vi "AlliGator Fit Termination Criteria & Quality Metrics Output String.vi"(8 "Error In":errorcluster, 9 "Fit Output":T5={"best nonlinear fit"=[], "best fit parameters"=[], "R^2"=0.0, "RMSE"=0.0, "error out"={"status"=FALSE, "code"=0, "source"=""}, "Fitting Method"=enum."Least Square", "number of function calls"=0, "number of iterations"=0, "covariance"=[], "Chi 2"=0.0, "DOF"=0, "Fit Convergence Criterion"=enum."Continue", "Fitting Algorithm"=enum."Levenberg-Marquardt", "Weighted Fit"=enum."Unweighted", "Gradient"=0.0, "|Delta Chi 2|"=0.0, "|Delta Chi 2|/Chi 2"=0.0, "Max |Delta a| /|a|"=0.0, "Lambda"=0.0, "RSS"=0.0, "AIC"=0.0, "BIC"=0.0, "Max number of function calls"=0, "Max number of iterations"=0, "IRF"={"X Array"=[], "Y Array"=[]}, "IRF Normalization Factor"=0.0, "Decay Normalization Factor"=0.0, "Number of offset fits"=0, "Weighted Chi2"=-1.0, "Unweighted Chi2"=-1.0}, 11 "Termination Criteria":T2) -> (0 "Error Out":errorcluster, 1 "Weighted Fit":T1, 3 "String":string)   [LabVIEW 2021, in "AlliGator Decay Fit.lvlib"]
doc: "Creates a string describing the fit termination criteria and quality metrics."
uses:
  AlliGator Decay Fit.lvlib
  Fits/Nonlinear Fit Method.ctl
  Fits/Fits.lvlib
  <vilib>/Analysis/Matrix/Datatypes/RealMatrix.ctl
  <vilib>/Analysis/Matrix/NI_Matrix.lvlib
  Fits/Convergence Criteria.ctl
  Fits/Non-linear Fitting Algorithm.ctl
  Fits/Non-linear Fit Output v4.ctl
  Graphs/XY Graph/XY Graph Plot Data.ctl
  Graphs/XY Graph/XY Graph Add-Ons.lvlib
  Fits/IRF(X)PSED/Fit Weights Type v2.ctl
panel:
  in  "Fitting Method":T3
  in  "Fitting Algorithm":T4
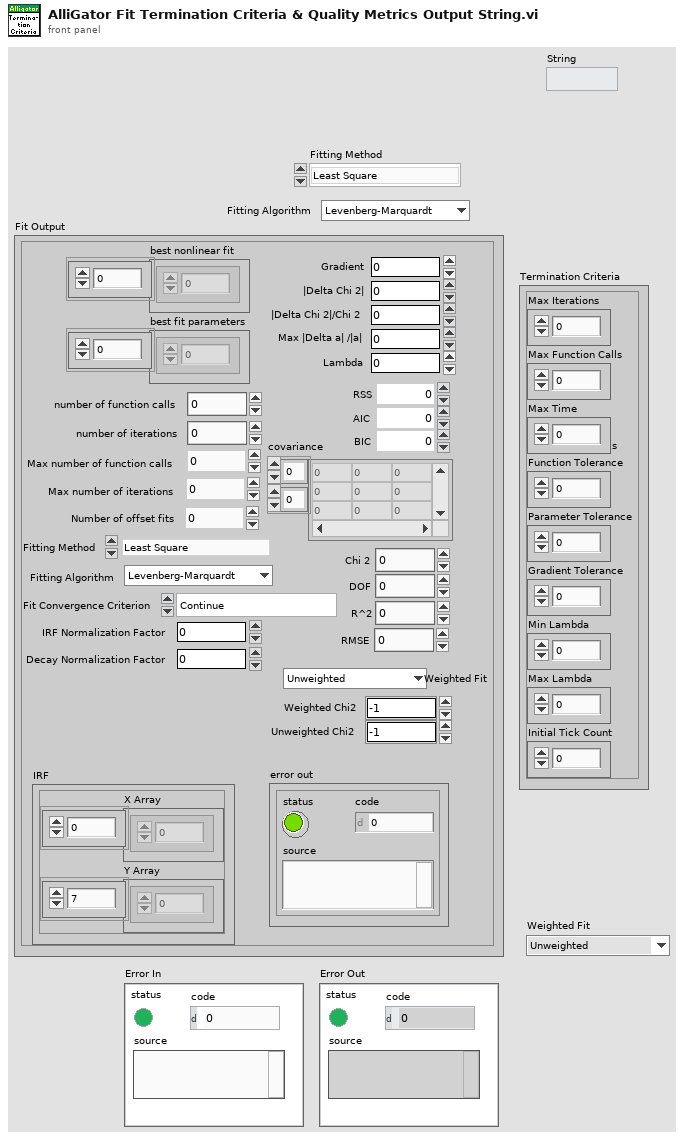
[diagram p1: front panel]
types:
  T1 = typedef "Fits.lvlib/Fit Weights Type v2.ctl" = enum16{"Unweighted", "1/Variance (Neyman)", "1/Variance (Pearson)", "Best of All"}
  T2 = cluster{"Max Iterations":i32, "Max Function Calls":i32, "Max Time":dbl[unit], "Function Tolerance":dbl, "Parameter Tolerance":dbl, "Gradient Tolerance":dbl, "Min Lambda":dbl, "Max Lambda":dbl, "Initial Tick Count":u32}
  T3 = typedef "Fits.lvlib/Nonlinear Fit Method.ctl" = enum16{"Least Square", "Least Absolute Residual", "Bisquare", "MLE"}
  T4 = typedef "Fits.lvlib/Non-linear Fitting Algorithm.ctl" = enum16{"Levenberg-Marquardt", "Trust-Region Dogleg"}
  T5 = typedef "Fits.lvlib/Non-linear Fit Output v4.ctl" = cluster{"best nonlinear fit":dbl[], "best fit parameters":dbl[], "R^2":dbl, "RMSE":dbl, "error out":errorcluster, "Fitting Method":T3, "number of function calls":i32, "number of iterations":i32, "covariance":T6, "Chi 2":dbl, "DOF":i32, "Fit Convergence Criterion":T7, "Fitting Algorithm":T4, "Weighted Fit":T1, "Gradient":dbl, "|Delta Chi 2|":dbl, "|Delta Chi 2|/Chi 2":dbl, "Max |Delta a| /|a|":dbl, "Lambda":dbl, "RSS":dbl, "AIC":dbl, "BIC":dbl, "Max number of function calls":i32, "Max number of iterations":i32, "IRF":T8, "IRF Normalization Factor":dbl, "Decay Normalization Factor":dbl, "Number of offset fits":i32, "Weighted Chi2":dbl, "Unweighted Chi2":dbl}
  T6 = typedef "NI_Matrix.lvlib/RealMatrix.ctl" = dbl[][]
  T7 = typedef "Fits.lvlib/Convergence Criteria.ctl" = enum16{"Continue", "Tolerances Exceeded", "Max Time Exceeded", "Max Iterations Exceeded", "Max Function Evaluations Exceeded", "Scale Range Exceeded"}
  T8 = typedef "XY Graph Add-Ons.lvlib/XY Graph Plot Data.ctl" = cluster{"X Array":dbl[], "Y Array":dbl[]}
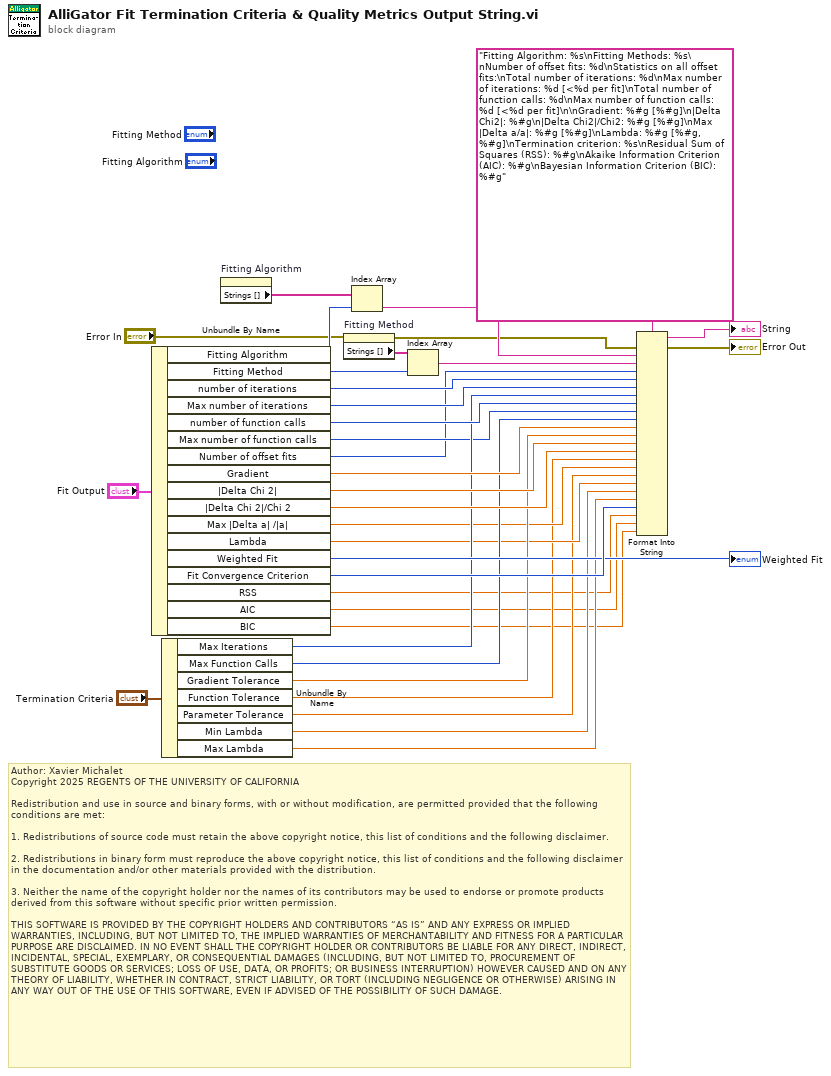
[diagram p0: block diagram]
diagram:
  # "Author: Xavier Michalet\nCopyright 2025 REGENTS OF THE UNIVERSITY OF CALIFORNIA\n\nRedistribution and use in source and binary forms, with or without modification, are permitted provided that the following conditions are met:\n\n1. Redistributions of source code must retain the above copyright notice, this list of conditions and the following disclaimer.\n\n2. Redistributions in binary form must reproduce the above copyright notice, this list of conditions and the following disclaimer in the documentation and/or other materials provided with the distribution.\n\n3. Neither the name of the copyright holder nor the names of its contributors may be used to endorse or promote products derived from this software without specific prior written permission.\n\nTHIS SOFTWARE IS PROVIDED BY THE COPYRIGHT HOLDERS AND CONTRIBUTORS “AS IS” AND ANY EXPRESS OR IMPLIED WARRANTIES, INCLUDING, BUT NOT LIMITED TO, THE IMPLIED WARRANTIES OF MERCHANTABILITY AND FITNESS FOR A PARTICULAR PURPOSE ARE DISCLAIMED. IN NO EVENT SHALL THE COPYRIGHT HOLDER OR CONTRIBUTORS BE LIABLE FOR ANY DIRECT, INDIRECT, INCIDENTAL, SPECIAL, EXEMPLARY, OR CONSEQUENTIAL DAMAGES (INCLUDING, BUT NOT LIMITED TO, PROCUREMENT OF SUBSTITUTE GOODS OR SERVICES; LOSS OF USE, DATA, OR PROFITS; OR BUSINESS INTERRUPTION) HOWEVER CAUSED AND ON ANY THEORY OF LIABILITY, WHETHER IN CONTRACT, STRICT LIABILITY, OR TORT (INCLUDING NEGLIGENCE OR OTHERWISE) ARISING IN ANY WAY OUT OF THE USE OF THIS SOFTWARE, EVEN IF ADVISED OF THE POSSIBILITY OF SUCH DAMAGE."
  n1 = Unbundle By Name("Fit Output") -> ("Fitting Algorithm"=w32:T4, "Fitting Method"=w26:T3, "number of iterations"=w27:i32, "Max number of iterations"=w3:i32, "number of function calls"=w28:i32, "Max number of function calls"=w2:i32, "Number of offset fits"=w1:i32, "Gradient"=w22:dbl, "|Delta Chi 2|"=w21:dbl, "|Delta Chi 2|/Chi 2"=w20:dbl, "Max |Delta a| /|a|"=w12:dbl, "Lambda"=w11:dbl, "Weighted Fit"=→"Weighted Fit":T1, "Fit Convergence Criterion"=w35:T7, "RSS"=w6:dbl, "AIC"=w5:dbl, "BIC"=w4:dbl)
  n2 = Unbundle By Name("Termination Criteria") -> ("Max Iterations"=w15:i32, "Max Function Calls"=w14:i32, "Gradient Tolerance"=w13:dbl, "Function Tolerance"=w10:dbl, "Parameter Tolerance"=w9:dbl, "Min Lambda"=w8:dbl, "Max Lambda"=w7:dbl)
  n3 = property on="Fitting Algorithm" class="Enum (strict)"() -> ("Strings []"=w23:string[])  [unwired: 2 in, 2 out]
  n4 = property on="Fitting Method" class="Enum (strict)"(error in="Error In") -> (error out=w18:errorcluster, "Strings []"=w24:string[])  [unwired: 1 in, 1 out]
  n5 = Index Array(array=w23, index=w32) -> (element=w33:string)
  n6 = Index Array(array=w24, index=w26) -> (element=w31:string)
  n7 = Format Into String(format string="Fitting Algorithm: %s\nFitting Methods: %s\nNumber of offset fits: %d\nStatistics on all offset fits:\nTotal number of iterations: %d\nMax number of iterations: %d [<%d per fit]\nTotal number of function calls: %d\nMax number of function calls: %d [<%d per fit]\n\nGradient: %#g [%#g]\n|Delta Chi2|: %#g\n|Delta Chi2|/Chi2: %#g [%#g]\nMax |Delta a/a|: %#g [%#g]\nLambda: %#g [%#g, %#g]\nTermination criterion: %s\nResidual Sum of Squares (RSS): %#g\nAkaike Information Criterion (AIC): %#g\nBayesian Information Criterion (BIC): %#g", error in=w18, w33, w31, w1, w27, w3, w15, w28, w2, w14, w22, w13, w21, w20, w10, w12, w9, w11, w8, w7, w35, w6, w5, w4) -> (resulting string=→"String":string, error out=→"Error Out":errorcluster)  [unwired: 1 in]
